vi "Read number_of_tactics.vi"(8 "error in (no error)":errorcluster, 11 "BallPlacementPasserRole in":refnum<class "BallPlacementPasserRole.lvclass">) -> (0 "error out":errorcluster, 2 "number_of_tactics":i32=3, 3 "BallPlacementPasserRole out":refnum<class "BallPlacementPasserRole.lvclass">)   [LabVIEW 2021, in "BallPlacementPasserRole.lvclass"]
uses:
  BallPlacementPasserRole.lvclass
  BallPlacementPasserRole.lvclass/BallPlacementPasserRole.ctl
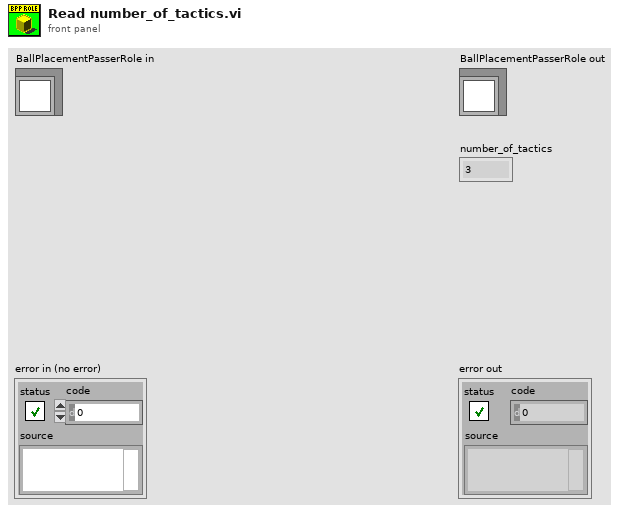
[diagram p1: front panel]
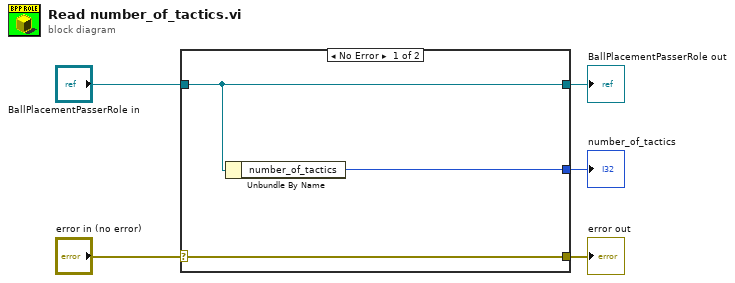
[diagram p0: block diagram]
diagram:
  n1 = case shown="No Error" "error in (no error)" {
    selector: "error in (no error)" -> [w8 w9]
    tunnel: [w8 w9] -> w4
    tunnel: [w7 w10] -> w2
    tunnel: "BallPlacementPasserRole in" -> [w7 w10]
    tunnel: [w6 _] -> w1
    frame No Error {
      n2 = Unbundle By Name(w7) -> ("number_of_tactics"=w6:i32)
    }
    frame Error {
    }
  }
  "error out" <- w4
  "BallPlacementPasserRole out" <- w2
  "number_of_tactics" <- w1
